vi "schoolZones.vi"(8 "School Zone Speed":dbl=0.1, 9 "Max. Speed":dbl=0.15, 10 "y":dbl=2635.374257532753, 11 "x":dbl=5713.048588279035) -> (3 "Speed":dbl=0.15)   [LabVIEW 2016]
panel:
  in  "robotDia":dbl=320.0
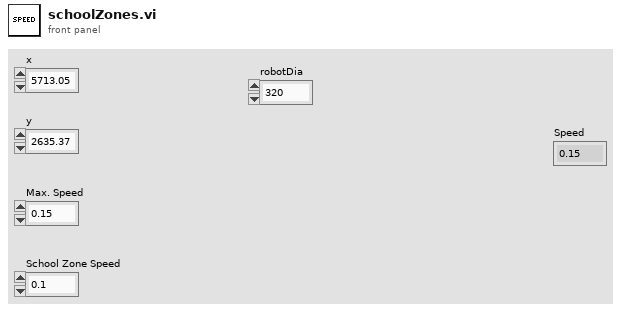
[diagram p1: front panel]
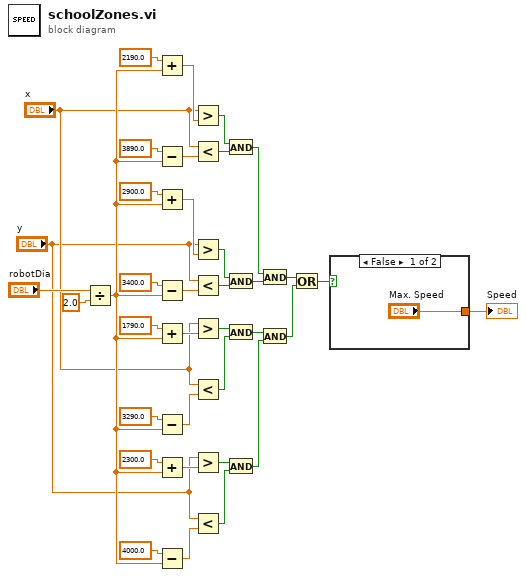
[diagram p0: block diagram]
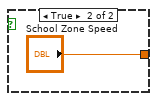
[diagram p2: hidden frame]
diagram:
  n1 = Divide(x="robotDia", y=2.0) -> (x/y=w6:dbl)
  n2 = Add(x=2190.0 ("y"), y=w6) -> (x+y=w23:dbl)
  n3 = Subtract(x=3890.0 ("y"), y=w6) -> (x-y=w26:dbl)
  n4 = Add(x=2900.0 ("y"), y=w6) -> (x+y=w21:dbl)
  n5 = Subtract(x=3400.0 ("y"), y=w6) -> (x-y=w27:dbl)
  n6 = Add(x=1790.0 ("y"), y=w6) -> (x+y=w9:dbl)
  n7 = Subtract(x=3290.0 ("y"), y=w6) -> (x-y=w12:dbl)
  n8 = Add(x=2300.0 ("y"), y=w6) -> (x+y=w7:dbl)
  n9 = Subtract(x=4000.0 ("y"), y=w6) -> (x-y=w13:dbl)
  n10 = Greater?(x="x", y=w23) -> (0:w32:bool)
  n11 = Less?(x="x", y=w26) -> (x < y?=w31:bool)
  n12 = Greater?(x="y", y=w21) -> (0:w35:bool)
  n13 = Less?(x="y", y=w27) -> (x < y?=w36:bool)
  n14 = Greater?(x="x", y=w9) -> (0:w16:bool)
  n15 = Less?(x="x", y=w12) -> (x < y?=w15:bool)
  n16 = Greater?(x="y", y=w7) -> (0:w19:bool)
  n17 = Less?(x="y", y=w13) -> (x < y?=w20:bool)
  n18 = And(x=w32, y=w31) -> (x .and. y?=w33:bool)
  n19 = And(x=w35, y=w36) -> (x .and. y?=w34:bool)
  n20 = And(x=w16, y=w15) -> (x .and. y?=w17:bool)
  n21 = And(x=w19, y=w20) -> (x .and. y?=w18:bool)
  n22 = And(x=w33, y=w34) -> (x .and. y?=w4:bool)
  n23 = And(x=w17, y=w18) -> (x .and. y?=w5:bool)
  n24 = Or(x=w4, y=w5) -> (x .or. y?=w3:bool)
  n25 = case shown="False" w3 {
    tunnel: ["Max. Speed" "School Zone Speed"] -> w37
    frame False {
    }
    frame True {
    }
  }
  "Speed" <- w37
